vi "while_v0_v3.vi"() -> ()   [LabVIEW 2010]
panel:
  in  "stop":bool
  out "Array":bool[](array[boolean])=[FALSE, TRUE, FALSE, FALSE, TRUE, FALSE, TRUE, TRUE]
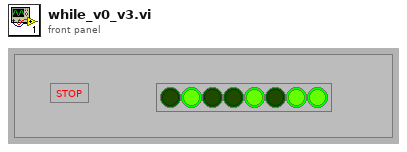
[diagram p1: front panel]
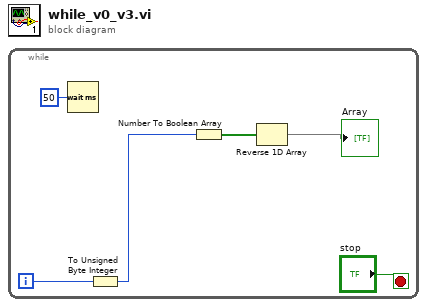
[diagram p0: block diagram]
diagram:
  n1 = while {
    i -> [w3]
    stop <- "stop" stop-if-true
    n2 = Wait (ms)(milliseconds to wait=u32 50) -> ()  [unwired: 1 out]
    n3 = To Unsigned Byte Integer(number=w3) -> (unsigned 8bit integer=w1:u8)
    n4 = Number To Boolean Array(number=w1) -> (Boolean array=w6:bool[])
    n5 = Reverse 1D Array(array=w6) -> (reversed array=→"Array":bool[])
  }
